vi "Color_detection.vi"   [LabVIEW 2019]
uses:
  Global Var.vi
types:
  T1 = typedef "IMAQ Image.ctl" = refnum<image>
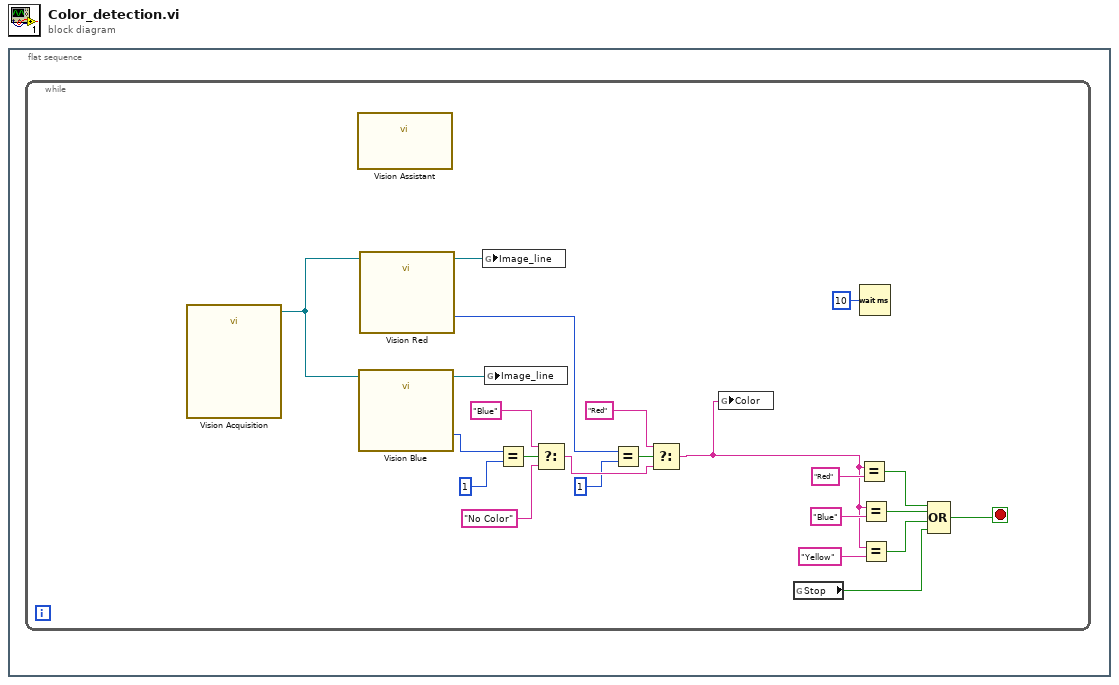
[diagram p0: block diagram]
diagram:
  n1 = flat-sequence {
    frame #0 {
      n2 = while {
        stop <- w2 stop-if-true
        n3 = call "Vision Acquisition"() -> ("Image Out"=w15:T1)  [unwired: 25 in, 2 out]
        n4 = call "Vision Assistant"() -> ()  [unwired: 12 in]
        n5 = call "Vision Blue"("Image In"=w15) -> ("Image Out"=w9:T1, "Number of Matches (Color Location 1)"=w10:i32)  [unwired: 24 in, 1 out]
        n6 = call "Vision Red"("Image In"=w15) -> ("Image Out"=w5:T1, "Number of Matches (Color Location 1)"=w4:i32)  [unwired: 24 in, 1 out]
        n7 = global write "Global Var.vi" "Image_line"(w5) -> ()
        n8 = global write "Global Var.vi" "Image_line"(w9) -> ()
        n9 = Equal?(x=w10, y=1) -> (x = y?=w13:bool)
        n10 = Select(t="Blue", s=w13, f="No Color") -> (s? t:f=w23:string)
        n11 = Equal?(x=w4, y=1) -> (x = y?=w7:bool)
        n12 = Select(t="Red", s=w7, f=w23) -> (s? t:f=w3:string)
        n13 = global write "Global Var.vi" "Color"(w3) -> ()
        n14 = global read "Global Var.vi" "Stop"() -> (w16:bool)
        n15 = Equal?(x=w3, y="Red") -> (x = y?=w19:bool)
        n16 = Wait (ms)(milliseconds to wait=u32 10) -> ()  [unwired: 1 out]
        n17 = Equal?(x=w3, y="Blue") -> (x = y?=w18:bool)
        n18 = Equal?(x=w3, y="Yellow") -> (x = y?=w17:bool)
        n19 = Compound Arithmetic op=OR(w19, w18, w17, w16) -> (w2:bool)
      }
    }
  }
